vi "Uniform White Noise (obs 90).vi"(2 "seed":i32=-1, 3 "amplitude":dbl=1.0 format="%0.2f", 4 "samples":i32=128) -> (0 "error":i32, 1 "uniform white noise":dbl[](array[numeric]))   [LabVIEW 2014, in "NI_AALBase.lvlib"]
doc: "The Uniform White Noise VI was rewritten in LabVIEW 2009. Replace this VI with a Uniform White Noise VI from the <B>Functions</B> palette to use the new functionality.\n\nGenerates a uniformly distributed, pseudorandom pattern whose values are in the range [-a:a], where a is the absolute value of <B>amplitude</B>.\n\nThe Uniform White Noise VI generates the pseudorandom sequence using a modified version of the Very-Long-Cycle random number generator algorithm. The pseudorandom number generator implements a triple-seeded linear congruential algorithm."
uses:
  NI_AALBase.lvlib
  lvanlys.dll
panel:
  # "Uniform White Noise"
  # "This VI is obsolete !!!\nYou should replace this VI in your diagram with the Uniform White Noise VI."
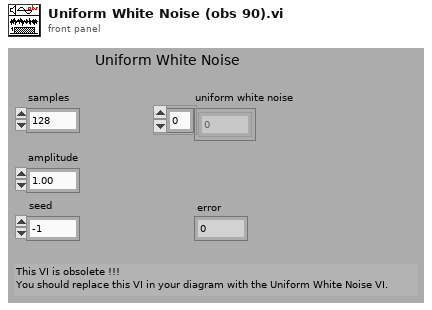
[diagram p1: front panel]
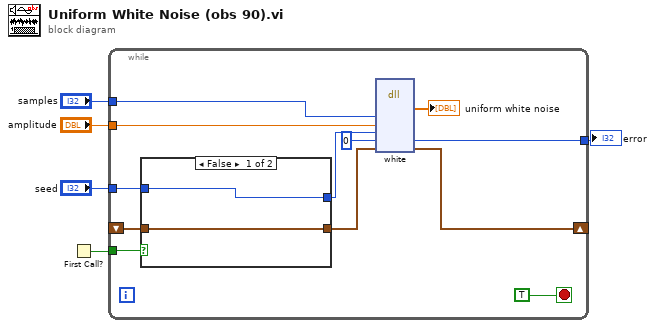
[diagram p0: block diagram]
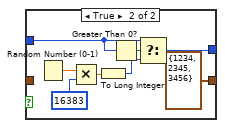
[diagram p2: hidden frame]
diagram:
  n1 = First Call?() -> (First Call?: T/F=w1:bool)
  n2 = while {
    tunnel: [w17] -> w5
    tunnel: "seed" -> [w10]
    tunnel: "amplitude" -> [w16]
    tunnel: "samples" -> [w15]
    shift-right: [w12] -> _
    shift-left: _ -> [w7]
    tunnel: w1 -> [w8]
    stop <- TRUE stop-if-true
    n3 = case shown="False" w8 {
      tunnel: w7 -> [w19 _]
      tunnel: [w19 cluster{"xSeed":i32, "ySeed":i32, "zSeed":i32} {"xSeed"=1234, "ySeed"=2345, "zSeed"=3456} ("RNGState")] -> w6
      tunnel: [w18 w25] -> w9
      tunnel: w10 -> [w18 w26]
      frame False {
      }
      frame True {
        n4 = Random Number (0-1)() -> (number: 0 to 1=w23:dbl)
        n5 = Multiply(x=w23, y=16383 ("x")) -> (x*y=w24:dbl)
        n6 = To Long Integer(number=w24) -> (32bit integer=w22:i32)
        n7 = Greater Than 0?(x=w26) -> (x > 0?=w27:bool)
        n8 = Select(t=w26, s=w27, f=w22) -> (s? t:f=w25:i32)
      }
    }
    n9 = dll-call lib="C:/Program Files (x86)/National Instruments/LabVIEW 2014/resource/lvanlys.*" fn="white"("size"=w15, "ampl"=w16, "theSeed"=w9, "dsperr"=0, "rng_state"=w6) -> ("uniform white noise"=→"uniform white noise":dbl[], "dsperr"=w17:i32, "rng_state"=w12:cluster{"xSeed":i32, "ySeed":i32, "zSeed":i32})  [unwired: 4 in, 6 out]
  }
  "error" <- w5
